vi "commpaser.vi"(6 "y_shift":dbl=1.75, 8 "large map":bool, 11 "Sensor [F12]":bool=TRUE) -> (0 "lane":dbl[][](array[numeric]), 1 "obs":dbl[][](array[numeric]), 2 "size(s)":i32, 3 "E-stop":bool, 4 "etc":dbl[][](array[numeric]))   [LabVIEW 2012]
uses:
  G_SEN.vi
  G_PATH.vi
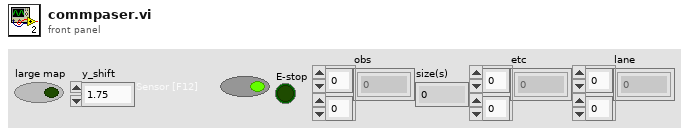
[diagram p1: front panel]
types:
  T1 = cluster{"global_x":sgl, " global_y":sgl, "yaw":sgl, "objCount":u16, "total":u16}
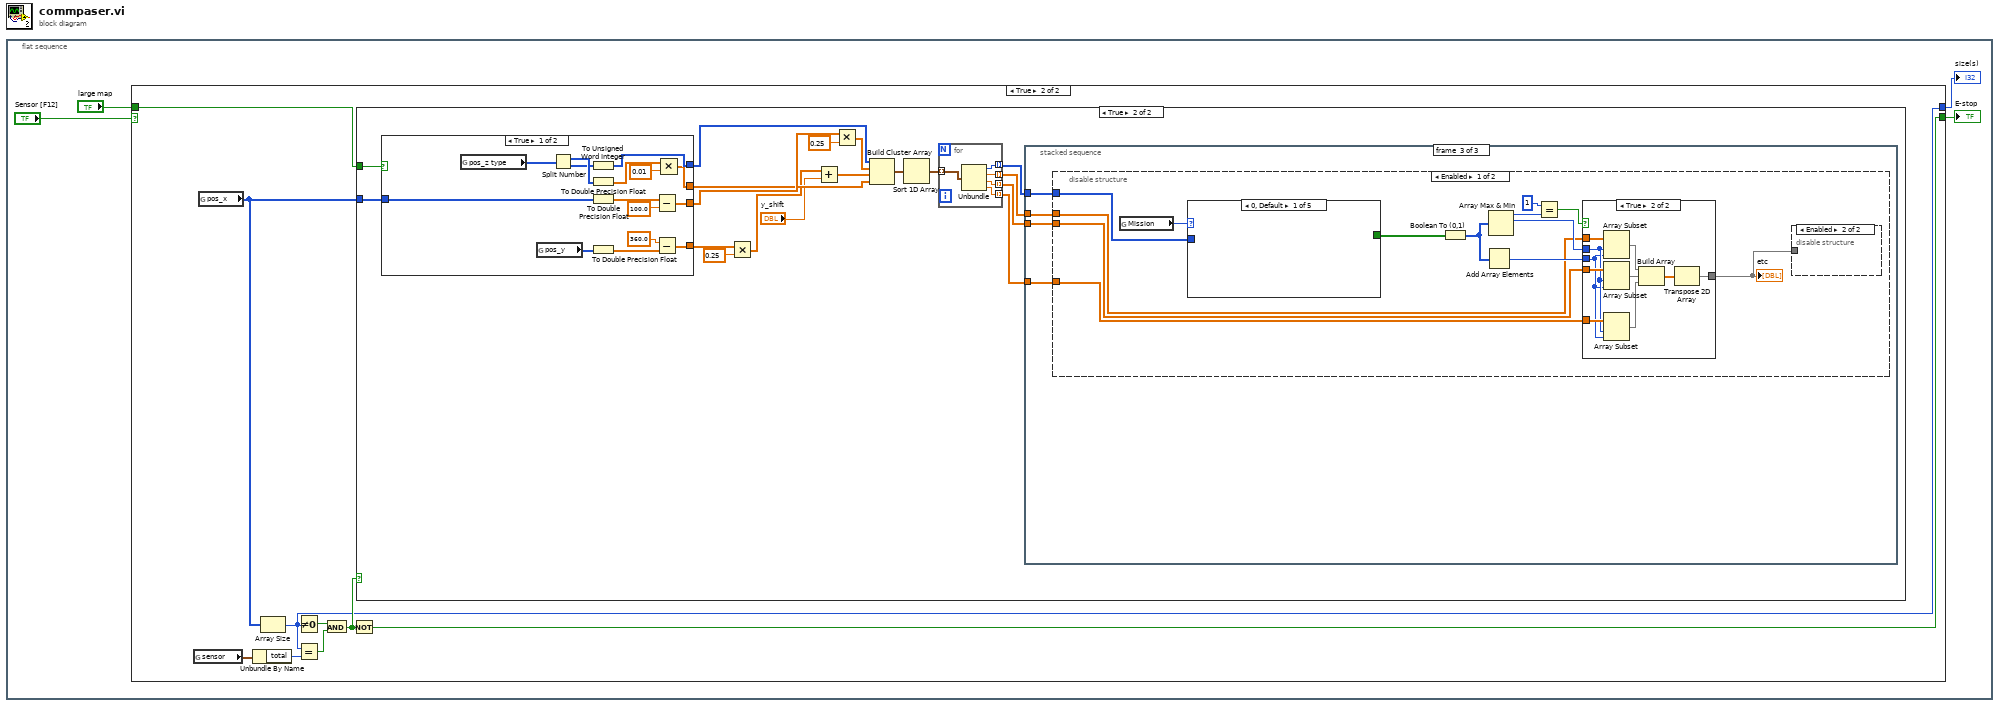
[diagram p0: block diagram]
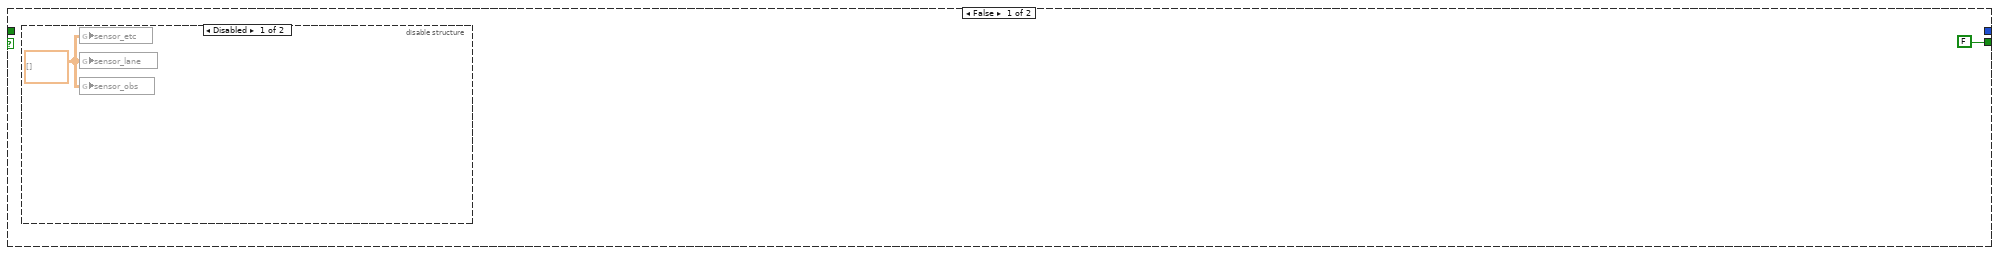
[diagram p2: hidden frame]
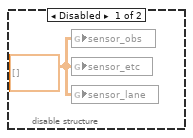
[diagram p5: hidden frame]
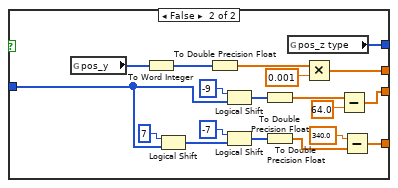
[diagram p6: hidden frame]
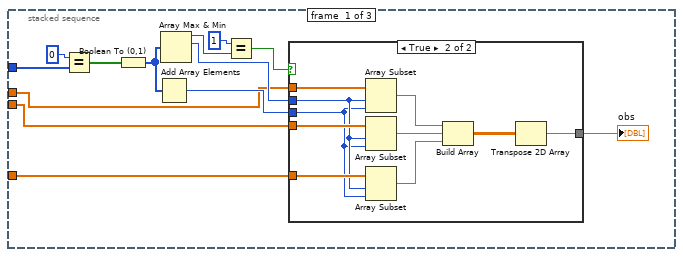
[diagram p7: hidden frame]
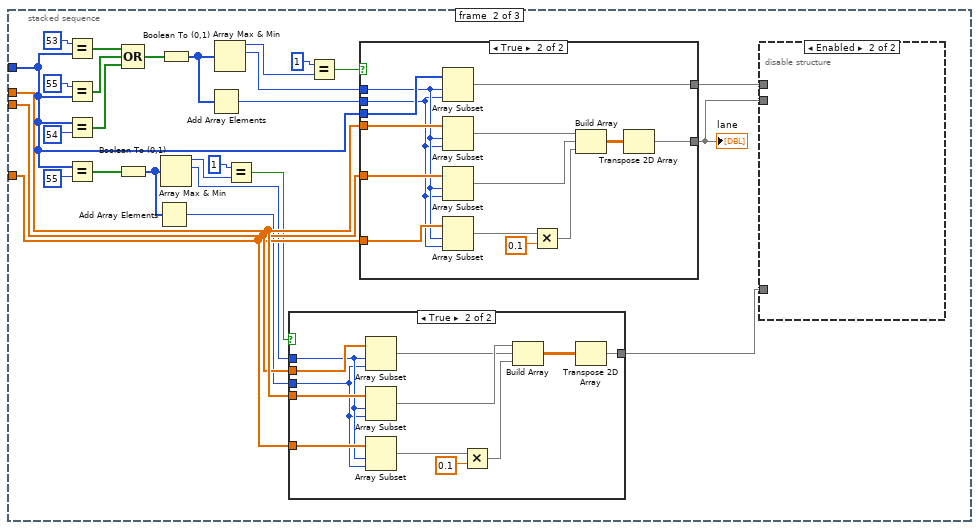
[diagram p9: hidden frame]
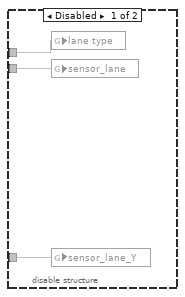
[diagram p10: hidden frame]
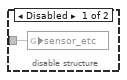
[diagram p13: hidden frame]
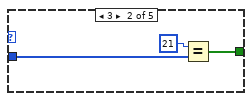
[diagram p14: hidden frame]
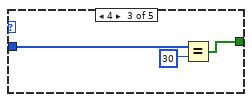
[diagram p15: hidden frame]
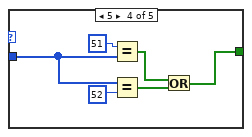
[diagram p16: hidden frame]
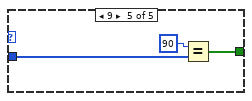
[diagram p17: hidden frame]
diagram:
  n1 = flat-sequence {
    frame #0 {
      n2 = case shown="True" "Sensor [F12]" {
        tunnel: [FALSE w13] -> w3
        tunnel: [_ w9] -> w2
        tunnel: "large map" -> [_ w7]
        frame False {
          n3 = disable-structure shown="Disabled" {
            frame Disabled {
              w6 = dbl[][] [] ("sensor_obs")
              n4 = global write "G_SEN.vi" "sensor_etc"(w6) -> ()
              n5 = global write "G_SEN.vi" "sensor_lane"(w6) -> ()
              n6 = global write "G_SEN.vi" "sensor_obs"(w6) -> ()
            }
            frame Enabled {
            }
          }
        }
        frame True {
          n7 = global read "G_SEN.vi" "sensor"() -> (w15:T1)
          n8 = global read "G_SEN.vi" "pos_x"() -> (w14:u16[])
          n9 = Unbundle By Name(w15) -> ("total"=w8:u16)
          n10 = Array Size(array=w14) -> (size(s)=w9:i32)
          n11 = Not Equal To 0?(x=w9) -> (x != 0?=w10:bool)
          n12 = Equal?(x=w9, y=w8) -> (x = y?=w11:bool)
          n13 = And(x=w10, y=w11) -> (x .and. y?=w12:bool)
          n14 = Not(x=w12) -> (.not. x?=w13:bool)
          n15 = case shown="True" w12 {
            tunnel: w14 -> [_ w25]
            tunnel: w7 -> [_ w21]
            frame False {
              n16 = disable-structure shown="Enabled" {
                frame Disabled {
                  w16 = dbl[][] [] ("sensor_obs")
                  n17 = global write "G_SEN.vi" "sensor_obs"(w16) -> ()
                  n18 = global write "G_SEN.vi" "sensor_etc"(w16) -> ()
                  n19 = global write "G_SEN.vi" "sensor_lane"(w16) -> ()
                }
                frame Enabled {
                }
              }
            }
            frame True {
              n20 = case shown="True" w21 {
                tunnel: [w47 w66] -> w33
                tunnel: [w44 w63] -> w30
                tunnel: w25 -> [w42 w60]
                tunnel: [w40 w58] -> w23
                tunnel: [w41 w50] -> w20
                frame True {
                  n21 = global read "G_SEN.vi" "pos_z type"() -> (w39:u16[])
                  n22 = global read "G_SEN.vi" "pos_y"() -> (w43:u16[])
                  n23 = Split Number(x=w39) -> (hi(x)=w38:u8[], lo(x)=w35:u8[])
                  n24 = To Unsigned Word Integer(number=w35) -> (unsigned 16bit integer=w41:u16[])
                  n25 = To Double Precision Float(number=w38) -> (double precision float=w36:dbl[])
                  n26 = To Double Precision Float(number=w42) -> (double precision float=w45:dbl[])
                  n27 = To Double Precision Float(number=w43) -> (double precision float=w48:dbl[])
                  n28 = Subtract(x=w45, y=100.0 ("x")) -> (x-y=w44:dbl[])
                  n29 = Subtract(x=360.0, y=w48) -> (x-y=w47:dbl[])
                  n30 = Multiply(x=w36, y=0.01) -> (x*y=w40:dbl[])
                }
                frame False {
                  n31 = global read "G_SEN.vi" "pos_y"() -> (w55:u16[])
                  n32 = To Word Integer(number=w55) -> (16bit integer=w57:i16[])
                  n33 = Logical Shift(y=i8 7, x=w60) -> (x << y=w53:u16[])
                  n34 = To Double Precision Float(number=w57) -> (double precision float=w56:dbl[])
                  n35 = Logical Shift(y=i8 -9, x=w60) -> (x << y=w61:u16[])
                  n36 = Logical Shift(y=i8 -7, x=w53) -> (x << y=w62:u16[])
                  n37 = To Double Precision Float(number=w61) -> (double precision float=w64:dbl[])
                  n38 = To Double Precision Float(number=w62) -> (double precision float=w67:dbl[])
                  n39 = global read "G_SEN.vi" "pos_z type"() -> (w50:u16[])
                  n40 = Multiply(x=w56, y=0.001) -> (x*y=w58:dbl[])
                  n41 = Subtract(x=w64, y=64.0 ("x")) -> (x-y=w63:dbl[])
                  n42 = Subtract(x=340.0, y=w67) -> (x-y=w66:dbl[])
                }
              }
              n43 = Multiply(x=w33, y=0.25) -> (x*y=w19:dbl[])
              n44 = Add(x=w19, y="y_shift") -> (x+y=w18:dbl[])
              n45 = Multiply(x=w30, y=0.25) -> (x*y=w34:dbl[])
              n46 = Build Cluster Array(w20, w34, w18, w23) -> (w29:cluster{"element":u16, dbl, dbl, dbl}[])
              n47 = Sort 1D Array(array=w29) -> (sorted array=w24:cluster{"element":u16, dbl, dbl, dbl}[])
              n48 = for {
                tunnel: w24 -> [w196] mode=indexing
                tunnel: [w195] -> w28 mode=indexing
                tunnel: [w194] -> w27 mode=indexing
                tunnel: [w193] -> w26 mode=indexing
                tunnel: [w192] -> w22 mode=indexing
                n49 = Unbundle(w196) -> ("element"=w195:u16, w194:dbl, w193:dbl, w192:dbl)
              }
              n50 = stacked-sequence {
                tunnel: w28 -> [w81 w100 w152]
                tunnel: w27 -> [w72 w104 w151]
                tunnel: w26 -> [w71 w103 w150]
                tunnel: w22 -> [w69 w102 w149]
                frame #0 {
                  n51 = Equal?(x=u16 0, y=w81) -> (x = y?=w79:bool[])
                  n52 = Boolean To (0,1)(Boolean=w79) -> (0, 1=w75:i16[])
                  n53 = Add Array Elements(numeric array=w75) -> (sum=w74:i16)
                  n54 = Array Max & Min(array=w75) -> (max value=w78:i16, max index (indices)=w73:i32)  [unwired: 2 out]
                  n55 = Equal?(x=i16 1, y=w78) -> (x = y?=w76:bool)
                  n56 = case shown="True" w76 {
                    tunnel: w74 -> [_ w83]
                    tunnel: w73 -> [_ w84]
                    tunnel: w72 -> [_ w91]
                    tunnel: w71 -> [_ w90]
                    tunnel: [_ w86] -> w70
                    tunnel: w69 -> [_ w85]
                    frame False {
                    }
                    frame True {
                      n57 = Array Subset(array=w91, index=w84, length=w83) -> (w88:dbl[])
                      n58 = Array Subset(array=w90, index=w84, length=w83) -> (w87:dbl[])
                      n59 = Array Subset(array=w85, index=w84, length=w83) -> (w82:dbl[])
                      n60 = Build Array(w88, w87, w82) -> (w89:dbl[][])
                      n61 = Transpose 2D Array(2D array=w89) -> (transposed array=w86:dbl[][])
                    }
                  }
                  "obs" <- w70
                }
                frame #1 {
                  n62 = Equal?(x=u16 53, y=w100) -> (x = y?=w106:bool[])
                  n63 = Equal?(x=u16 55, y=w100) -> (x = y?=w109:bool[])
                  n64 = Equal?(x=w100, y=u16 54) -> (x = y?=w110:bool[])
                  n65 = Equal?(x=w100, y=u16 55) -> (x = y?=w96:bool[])
                  n66 = Boolean To (0,1)(Boolean=w96) -> (0, 1=w99:i16[])
                  n67 = Compound Arithmetic op=OR(w106, w109, w110) -> (w108:bool[])
                  n68 = Add Array Elements(numeric array=w99) -> (sum=w93:i16)
                  n69 = Boolean To (0,1)(Boolean=w108) -> (0, 1=w115:i16[])
                  n70 = Array Max & Min(array=w99) -> (max value=w97:i16, max index (indices)=w94:i32)  [unwired: 2 out]
                  n71 = Add Array Elements(numeric array=w115) -> (sum=w114:i16)
                  n72 = Array Max & Min(array=w115) -> (max value=w118:i16, max index (indices)=w113:i32)  [unwired: 2 out]
                  n73 = Equal?(x=i16 1, y=w97) -> (x = y?=w95:bool)
                  n74 = case shown="True" w95 {
                    tunnel: w93 -> [_ w125]
                    tunnel: w94 -> [_ w126]
                    tunnel: w104 -> [_ w134]
                    tunnel: w103 -> [_ w133]
                    tunnel: [_ w124] -> w92
                    tunnel: w102 -> [_ w130]
                    frame False {
                    }
                    frame True {
                      n75 = Array Subset(array=w133, index=w126, length=w125) -> (w131:dbl[])
                      n76 = Array Subset(array=w134, index=w126, length=w125) -> (w132:dbl[])
                      n77 = Array Subset(array=w130, index=w126, length=w125) -> (w129:dbl[])
                      n78 = Multiply(x=w129, y=0.1) -> (x*y=w127:dbl[])
                      n79 = Build Array(w132, w131, w127) -> (w123:dbl[][])
                      n80 = Transpose 2D Array(2D array=w123) -> (transposed array=w124:dbl[][])
                    }
                  }
                  n81 = Equal?(x=i16 1, y=w118) -> (x = y?=w116:bool)
                  n82 = case shown="True" w116 {
                    tunnel: w114 -> [_ w136]
                    tunnel: w113 -> [_ w137]
                    tunnel: w104 -> [_ w148]
                    tunnel: w103 -> [_ w147]
                    tunnel: [_ w143] -> w112
                    tunnel: w102 -> [_ w142]
                    tunnel: w100 -> [_ w138]
                    tunnel: [_ w135] -> w105
                    frame False {
                    }
                    frame True {
                      n83 = Array Subset(array=w138, index=w137, length=w136) -> (w135:u16[])
                      n84 = Array Subset(array=w148, index=w137, length=w136) -> (w145:dbl[])
                      n85 = Array Subset(array=w147, index=w137, length=w136) -> (w144:dbl[])
                      n86 = Array Subset(array=w142, index=w137, length=w136) -> (w141:dbl[])
                      n87 = Multiply(x=w141, y=0.1) -> (x*y=w139:dbl[])
                      n88 = Build Array(w145, w144, w139) -> (w146:dbl[][])
                      n89 = Transpose 2D Array(2D array=w146) -> (transposed array=w143:dbl[][])
                    }
                  }
                  "lane" <- w112
                  n90 = disable-structure shown="Enabled" {
                    disable-tunnel: w112 -> [w122 _]
                    disable-tunnel: w105 -> [w121 _]
                    disable-tunnel: w92 -> [w120 _]
                    frame Disabled {
                      n91 = global write "G_SEN.vi" "lane type"(w121) -> ()
                      n92 = global write "G_SEN.vi" "sensor_lane"(w122) -> ()
                      n93 = global write "G_SEN.vi" "sensor_lane_Y"(w120) -> ()
                    }
                    frame Enabled {
                    }
                  }
                }
                frame #2 {
                  n94 = disable-structure shown="Enabled" {
                    disable-tunnel: w152 -> [w154 _]
                    disable-tunnel: w151 -> [w158 _]
                    disable-tunnel: w150 -> [w157 _]
                    disable-tunnel: w149 -> [w156 _]
                    frame Enabled {
                      n95 = global read "G_PATH.vi" "Mission"() -> (w153:i32)
                      n96 = case shown="0, Default" w153 {
                        tunnel: [_ w167 w170 w173 w181] -> w155
                        tunnel: w154 -> [_ w168 w172 w176 w180]
                        frame 0, Default {
                        }
                        frame 3 {
                          n97 = Equal?(x=u16 21, y=w168) -> (x = y?=w167:bool[])
                        }
                        frame 4 {
                          n98 = Equal?(x=w172, y=u16 30) -> (x = y?=w170:bool[])
                        }
                        frame 5 {
                          n99 = Equal?(x=u16 51, y=w176) -> (x = y?=w174:bool[])
                          n100 = Equal?(x=w176, y=u16 52) -> (x = y?=w175:bool[])
                          n101 = Or(x=w174, y=w175) -> (x .or. y?=w173:bool[])
                        }
                        frame 9 {
                          n102 = Equal?(x=u16 90, y=w180) -> (x = y?=w181:bool[])
                        }
                      }
                      n103 = Boolean To (0,1)(Boolean=w155) -> (0, 1=w162:i16[])
                      n104 = Add Array Elements(numeric array=w162) -> (sum=w163:i16)
                      n105 = Array Max & Min(array=w162) -> (max value=w159:i16, max index (indices)=w164:i32)  [unwired: 2 out]
                      n106 = Equal?(x=i16 1, y=w159) -> (x = y?=w161:bool)
                      n107 = case shown="True" w161 {
                        tunnel: w163 -> [_ w183]
                        tunnel: w164 -> [_ w184]
                        tunnel: w158 -> [_ w191]
                        tunnel: w157 -> [_ w190]
                        tunnel: [_ w186] -> w165
                        tunnel: w156 -> [_ w185]
                        frame False {
                        }
                        frame True {
                          n108 = Array Subset(array=w191, index=w184, length=w183) -> (w188:dbl[])
                          n109 = Array Subset(array=w190, index=w184, length=w183) -> (w187:dbl[])
                          n110 = Array Subset(array=w185, index=w184, length=w183) -> (w182:dbl[])
                          n111 = Build Array(w188, w187, w182) -> (w189:dbl[][])
                          n112 = Transpose 2D Array(2D array=w189) -> (transposed array=w186:dbl[][])
                        }
                      }
                      "etc" <- w165
                      n113 = disable-structure shown="Enabled" {
                        disable-tunnel: w165 -> [w166 _]
                        frame Disabled {
                          n114 = global write "G_SEN.vi" "sensor_etc"(w166) -> ()
                        }
                        frame Enabled {
                        }
                      }
                    }
                    frame Disabled {
                    }
                  }
                }
              }
            }
          }
        }
      }
      "E-stop" <- w3
      "size(s)" <- w2
    }
  }
